vi "build_cmd_packet.vi"(10 "message":string) -> (2 "command packet":string)   [LabVIEW 2018]
doc: "Build the command packet from the message. The format for the command packet is <length><message><checksum>."
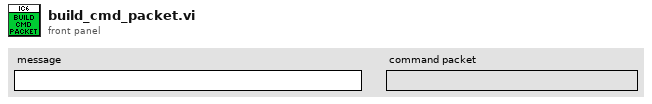
[diagram p1: front panel]
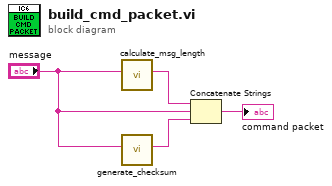
[diagram p0: block diagram]
diagram:
  n1 = call "calculate_msg_length.vi"("message"="message") -> ("length"=w3:string)  [unwired: 10 in]
  n2 = call "generate_checksum.vi"("message"="message") -> ("checksum"=w1:string)  [unwired: 10 in]
  n3 = Concatenate Strings(w3, "message", w1) -> (→"command packet":string)
